vi "GUI_SubVi.vi"(9 "Mode":bool, 10 "Time":dbl, 11 "Numeric":dbl) -> (3 "f":dbl)   [LabVIEW 2021]
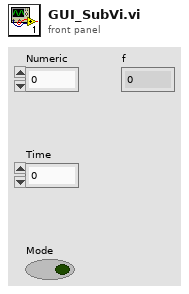
[diagram p1: front panel]
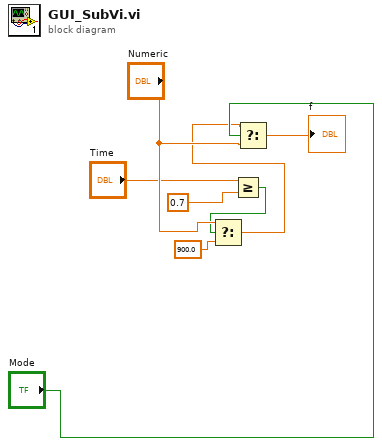
[diagram p0: block diagram]
diagram:
  n1 = Greater Or Equal?(x="Time", y=0.7) -> (x >= y?=w1:bool)
  n2 = Select(t="Numeric", s=w1, f=900.0) -> (s? t:f=w6:dbl)
  n3 = Select(t=w6, s="Mode", f="Numeric") -> (s? t:f=→"f":dbl)
